vi "On trigger signal acquisition.vi"() -> ()   [LabVIEW 2010]
doc: "This example shows how to acquire 16k samples of signal on fast analog inputs. Signal will be acquired when the internal trigger condition is meet. Time length of the acquired signal depends on the time scale of a buffer that can be set with a decimation factor. Decimations and time scales of a buffer are given in the table below. Voltage range of fast analog inputs on the Red Pitaya depends on gain setting that can be set by jumpers. HV setting is for input range to ±20V, while LV sets input range to ±1V."
uses:
  RedPitaya.lvlib
panel:
  in  "Gain Voltage":enum16{"Low voltage", "High voltage"}(ring)
  in  "Trigger Level (0 V)":dbl=1.1 min=-20.0 max=20.1
  in  "Delay (# Samples)":i32
  in  "Decimation":u32(ring)=8 items=["65536"=65536, "8192"=8192, "1024"=1024, "64"=64, "8"=8, "1"=1]
  in  "IP address":string="192.168.178.107"
  out "Waveform Graph":dbl[](graph)
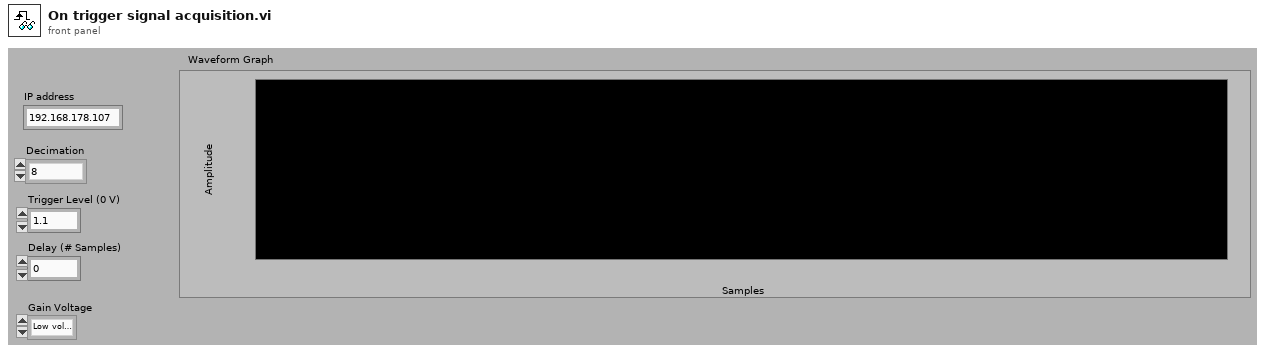
[diagram p1: front panel]
types:
  T1 = enum16{"Disabled", "Now", "Ch1 positive edge", "Ch1 negative edge", "Ch2 positive edge", "Ch2 negative edge", "external positive ege", "external negative edge", "AWG positive edge", "AWG negative edge"}
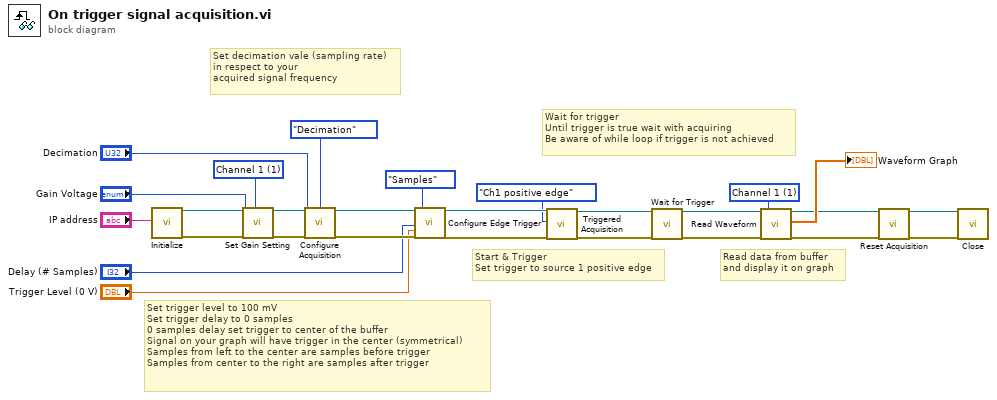
[diagram p0: block diagram]
diagram:
  w2 = u16 1 items=["Channel 1"=1, "Channel 2"=2] ("Channel #")
  w27 = u16 1 items=["Channel 1"=1, "Channel 2"=2] ("Channel (1|2)")
  # "Read data from buffer\nand display it on graph"
  # "Wait for trigger\nUntil trigger is true wait with acquiring\nBe aware of while loop if trigger is not achieved"
  # "Start & Trigger\nSet trigger to source 1 positive edge"
  # "Set trigger level to 100 mV\nSet trigger delay to 0 samples\n0 samples delay set trigger to center of the buffer\nSignal on your graph will have trigger in the center (symmetrical)\nSamples from left to the center are samples before trigger \nSamples from center to the right are samples after trigger"
  # "Set decimation vale (sampling rate)\nin respect to your\nacquired signal frequency"
  n1 = call "Initialize.vi"("IP address"="IP address") -> ("RedPitaya connection out"=w5:refnum<k5>, "error out"=w6:errorcluster)  [unwired: 17 in]
  n2 = call "Set Gain Setting.vi"("RedPitaya connection in"=w5, "Gain Voltage"="Gain Voltage", "error in"=w6, "Channel #"=w2) -> ("RedPitaya connection out"=w3:refnum<k5>, "error out"=w4:errorcluster)  [unwired: 14 in]
  n3 = call "Configure Acquisition.vi"("RedPitaya connection in"=w3, "Decimation/Sampling Rate"=enum16{"", "Sampling rate", "Decimation"}."Decimation", "Decimation"="Decimation", "error in"=w4) -> ("RedPitaya connection out"=w14:refnum<k5>, "error out"=w13:errorcluster)  [unwired: 14 in]
  n4 = call "Configure Edge Trigger.vi"("RedPitaya connection in"=w14, "Trigger Delay mode"=enum16{"", "Samples", "Nanoseconds"}."Samples", "Delay (# Samples)"="Delay (# Samples)", "Trigger Level (0 V)"="Trigger Level (0 V)", "error in"=w13) -> ("RedPitaya connection out"=w25:refnum<k5>, "error out"=w24:errorcluster)  [unwired: 13 in]
  n5 = call "Triggered Acquisition.vi"("RedPitaya TCP connection in"=w25, "Trigger Mode"=T1."Ch1 positive edge", "error in"=w24) -> ("RedPitaya TCP connection out"=w22:refnum<k5>, "error out"=w19:errorcluster)  [unwired: 15 in]
  n6 = call "Wait for Trigger.vi"("RedPitaya TCP connection in"=w22, "error in"=w19) -> ("RedPitaya TCP connection out"=w21:refnum<k5>, "error out"=w20:errorcluster)  [unwired: 16 in]
  n7 = call "Read Waveform.vi"("RedPitaya TCP Connection in"=w21, "error in"=w20, "Channel #"=w27) -> ("RedPitaya TCP Connection out"=w18:refnum<k5>, "Measurement Array"=→"Waveform Graph":dbl[], "error out"=w16:errorcluster)  [unwired: 14 in]
  n8 = call "Reset Acquisition.vi"("RedPitaya connection in"=w18, "error in"=w16) -> ("RedPitaya connection out"=w17:refnum<k5>, "error out"=w15:errorcluster)  [unwired: 16 in]
  n9 = call "Close.vi"("RedPitaya connection in"=w17, "error in"=w15) -> ()  [unwired: 17 in, 1 out]
